vi "UnProject.vi"(8 "error in":errorcluster, 10 "winCoords in":T1, 11 "class data in":refnum<class "SceneRoot.lvclass">) -> (0 "error out":errorcluster, 2 "sceneCoords out":T2, 3 "class data out":refnum<class "SceneRoot.lvclass">)   [LabVIEW 2010, in "RenderBase.lvlib" / "SceneRoot.lvclass"]
doc: "Converts window coordinates into scene coordinates."
uses:
  SceneRoot.lvclass
  <vilib>/Utility/miscctls.llb/LV3DPointTypeDef.ctl
  <vilib>/Utility/miscctls.llb/LVPoint32TypeDef.ctl
  SceneRoot.lvclass/SceneRoot.ctl
  <vilib>/Analysis/baseanly.llb/Real A x B.vi
  <vilib>/Analysis/baseanly.llb/Real Inverse Matrix.vi
  <vilib>/Analysis/baseanly.llb/A x Vector.vi
  <vilib>/Analysis/NI_AALBase.lvlib
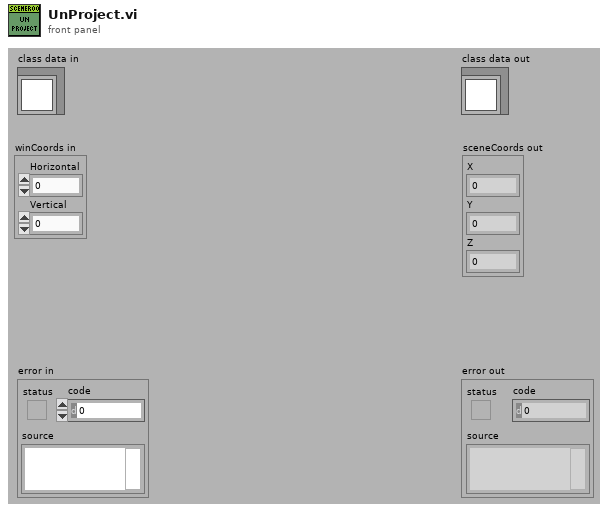
[diagram p1: front panel]
types:
  T1 = typedef "LVPoint32TypeDef.ctl" = cluster{"Horizontal":i32, "Vertical":i32}
  T2 = typedef "LV3DPointTypeDef.ctl" = cluster{"X":sgl, "Y":sgl, "Z":sgl}
  T3 = typedef "NI_Matrix.lvlib/RealMatrix.ctl" = dbl[][]
  T4 = cluster{"A x Vector[0]":dbl, "A x Vector[1]":dbl, "A x Vector[2]":dbl}
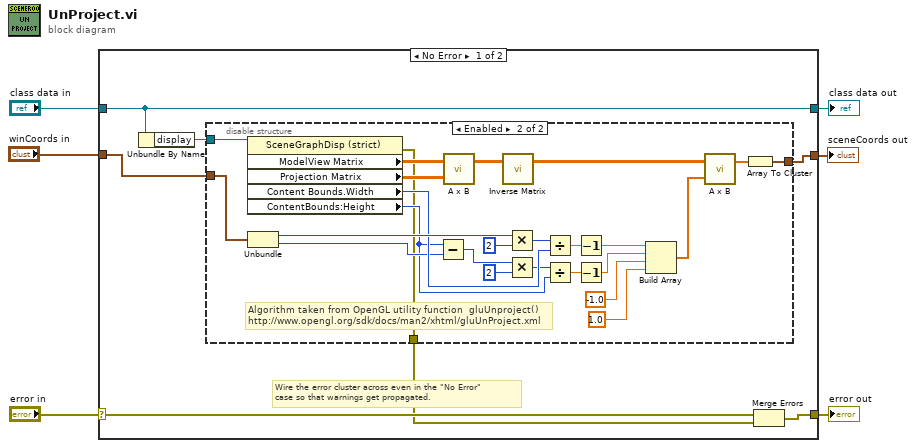
[diagram p0: block diagram]
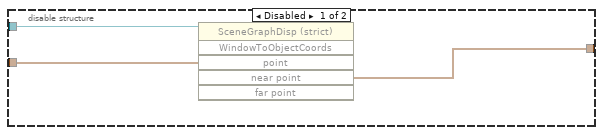
[diagram p2: hidden frame]
diagram:
  n1 = case shown="No Error" "error in" {
    selector: "error in" -> [w13 w43]
    tunnel: [w8 w43] -> w5
    tunnel: [w12 w42] -> w3
    tunnel: "class data in" -> [w12 w42]
    tunnel: "winCoords in" -> [w10 _]
    tunnel: [w9 _] -> w1
    frame No Error {
      # "Wire the error cluster across even in the \"No Error\"\ncase so that warnings get propagated."
      n2 = Unbundle By Name(w12) -> ("display"=w11:refnum<vi>)
      n3 = disable-structure shown="Enabled" {
        disable-tunnel: w11 -> [w16 w41]
        disable-tunnel: [w15 w39] -> w9
        disable-tunnel: w10 -> [w14 w40]
        disable-tunnel: [_ w17] -> w7
        frame Disabled {
          n4 = invoke on="Invoke Node" class="SceneGraphDisp (strict)" method="WindowToObjectCoords"(reference=w16, "point"=w14) -> ("near point"=w15:T2)  [unwired: 4 in, 5 out]
        }
        frame Enabled {
          # "Algorithm taken from OpenGL utility function  gluUnproject()\nhttp://www.opengl.org/sdk/docs/man2/xhtml/gluUnProject.xml"
          n5 = property class="SceneGraphDisp (strict)"(reference=w41) -> (error out=w17:errorcluster, "ModelView Matrix"=w31:sgl[][], "Projection Matrix"=w30:sgl[][], "Content Bounds.Width"=w37:u32, "ContentBounds:Height"=w28:u32)  [unwired: 1 in, 1 out]
          n6 = Unbundle(w40) -> ("Horizontal"=w38:i32, "Vertical"=w36:i32)
          n7 = Subtract(x=w28, y=w36) -> (x-y=w29:u32)
          n8 = call-poly <vilib>:"A x B.vi"("B"=w30, "A"=w31) -> ("A x B"=w35:T3)  [unwired: 1 out]
          n9 = call-poly <vilib>:"Inverse Matrix.vi"("Input Matrix"=w35) -> ("Inverse Matrix"=w33:T3)  [unwired: 1 in, 1 out]
          n10 = Multiply(x=w38, y=2) -> (x*y=w25:i32)
          n11 = Multiply(x=w29, y=u32 2) -> (x*y=w24:u32)
          n12 = Divide(x=w25, y=w37) -> (x/y=w23:dbl)
          n13 = Divide(x=w24, y=w28) -> (x/y=w22:dbl)
          n14 = Decrement(x=w23) -> (x-1=w21:dbl)
          n15 = Decrement(x=w22) -> (x-1=w20:dbl)
          n16 = Build Array(w21, w20, -1.0 ("element"), 1.0 ("element")) -> (w32:dbl[])
          n17 = call-poly <vilib>:"A x B.vi"("Vector"=w32, "A"=w33) -> ("A x Vector"=w34:dbl[])  [unwired: 1 out]
          n18 = Array To Cluster(array=w34) -> (cluster=w39:T4)
        }
      }
      n19 = Merge Errors(w13, w7) -> (w8:errorcluster)
    }
    frame Error {
    }
  }
  "error out" <- w5
  "class data out" <- w3
  "sceneCoords out" <- w1
